vi "Data Sensor.vi"(0 "VISA resource name":refnum<visa-resource-name>, 5 "Input (0:All)":u16(ring) items=["All Inputs", "1", "2", "3", "4", "5", "6", "7", "8"], 7 "Data Source (0:Kelvin)":u16(ring) items=["Kelvin", "Celsius", "Sensor Units", "Linear Data"], 11 "error in (no error)":errorcluster) -> (1 "Input 1":dbl min=-9999.9 max=9999.9 step=0.0001 format="%.4f", 2 "Input 2":dbl min=-9999.9 max=9999.9 step=0.0001 format="%.4f", 3 "Input 3":dbl min=-9999.9 max=9999.9 step=0.0001 format="%.4f", 4 "VISA resource name out":refnum<visa-resource-name>, 6 "Input 4":dbl min=-9999.9 max=9999.9 step=0.0001 format="%.4f", 8 "Input 5":dbl min=-9999.9 max=9999.9 step=0.0001 format="%.4f", 10 "Input 6":dbl min=-9999.9 max=9999.9 step=0.0001 format="%.4f", 13 "Input 8":dbl min=-9999.9 max=9999.9 step=0.0001 format="%.4f", 14 "Input 7":dbl min=-9999.9 max=9999.9 step=0.0001 format="%.4f", 15 "error out":errorcluster)   [LabVIEW 2017, in "Lake Shore Cryotronics 218.lvlib"]
doc: "This VI reads the sensor data from all 8 of the 218's inputs. All inputs may be read with one query, this should be done to achieve the maximum reading rate of 16 rdgs/sec of all inputs. This VI can also be configured to read only one input at a time."
uses:
  Lake Shore Cryotronics 218.lvlib
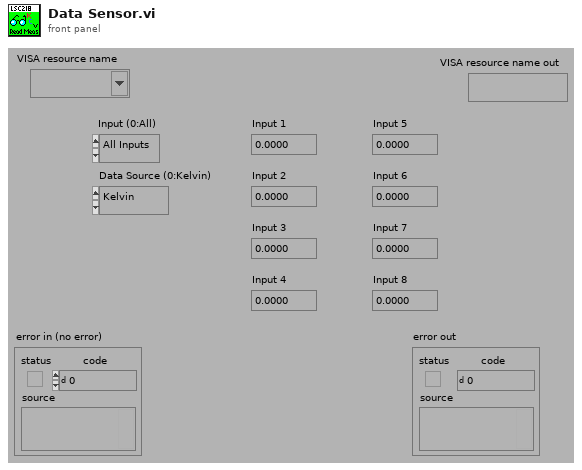
[diagram p1: front panel]
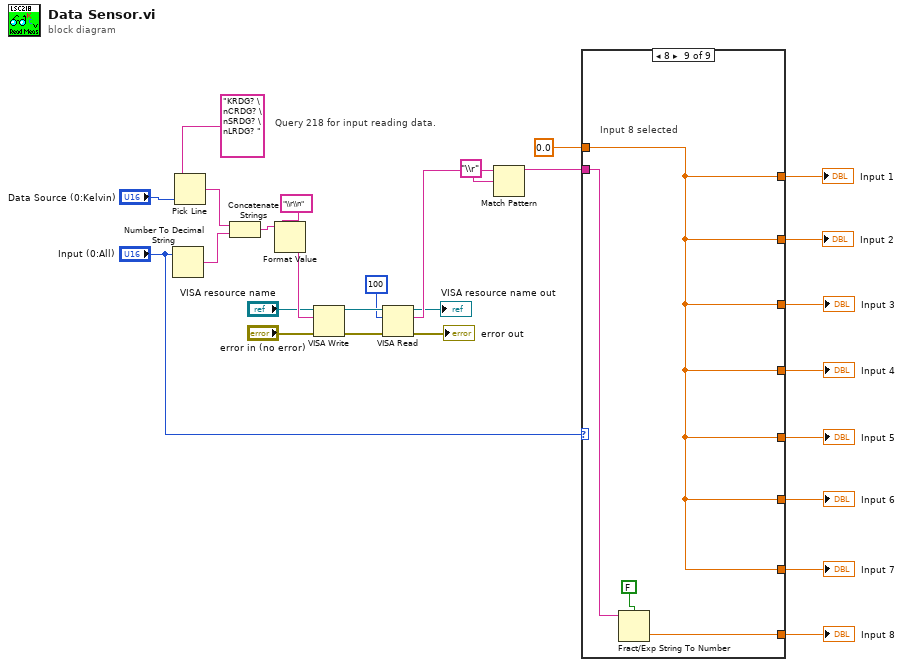
[diagram p0: block diagram]
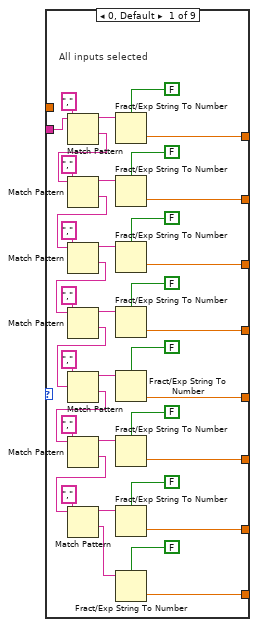
[diagram p2: hidden frame]
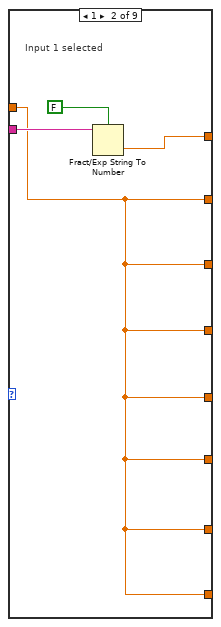
[diagram p3: hidden frame]
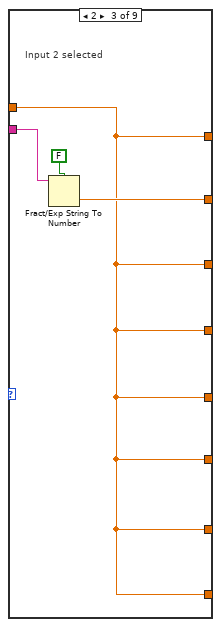
[diagram p4: hidden frame]
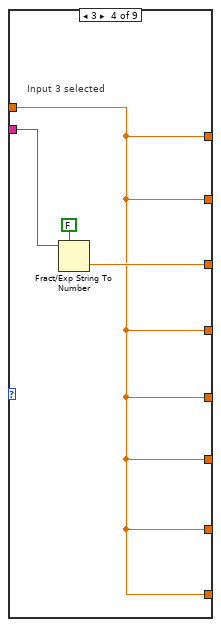
[diagram p5: hidden frame]
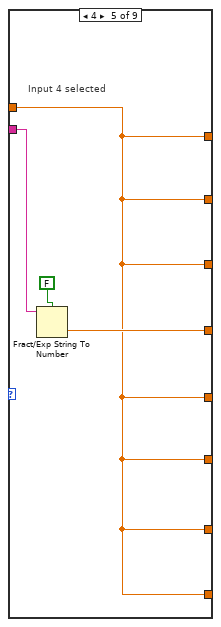
[diagram p6: hidden frame]
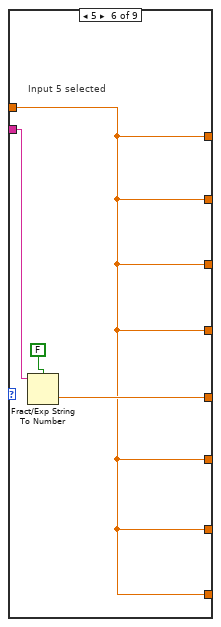
[diagram p7: hidden frame]
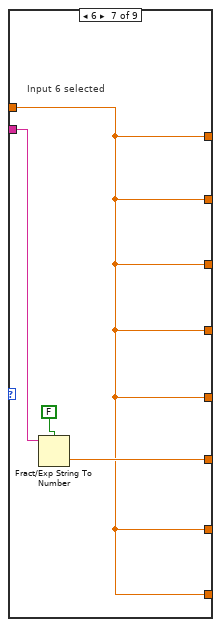
[diagram p8: hidden frame]
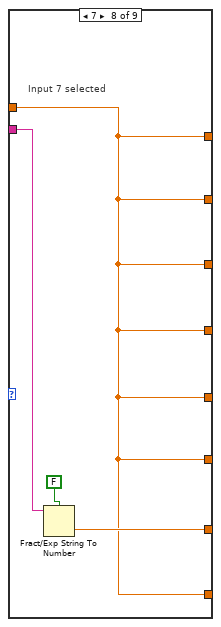
[diagram p9: hidden frame]
diagram:
  # "Query 218 for input reading data."
  n1 = Number To Decimal String(number="Input (0:All)") -> (decimal integer string=w19:string)  [unwired: 1 in]
  n2 = Pick Line(multi-line string="KRDG? \nCRDG? \nSRDG? \nLRDG? ", line index="Data Source (0:Kelvin)") -> (output string=w20:string)  [unwired: 1 in]
  n3 = Concatenate Strings(w20, w19) -> (w5:string)
  n4 = Format Value(string ("")=w5, format string="\\r\\n") -> (output string=w6:string)  [unwired: 1 in]
  n5 = VISA Write(VISA resource name="VISA resource name", write buffer=w6, error in (no error)="error in (no error)") -> (VISA resource name out=w27:refnum<visa-resource-name>, error out=w26:errorcluster)  [unwired: 1 out]
  n6 = VISA Read(VISA resource name=w27, byte count=100, error in (no error)=w26) -> (VISA resource name out=→"VISA resource name out":refnum<visa-resource-name>, read buffer=w24:string, error out=→"error out":errorcluster)  [unwired: 1 out]
  n7 = Match Pattern(string=w24, regular expression="\\r") -> (before substring=w17:string)  [unwired: 1 in, 3 out]
  n8 = case shown="8" "Input (0:All)" {
    tunnel: w17 -> [w65 w69 w73 w77 w81 w85 w89 w93 w97]
    tunnel: [w62 w68 w71 w75 w79 w83 w87 w91 w95] -> w16
    tunnel: [w58 w67 w72 w75 w79 w83 w87 w91 w95] -> w15
    tunnel: [w54 w67 w71 w76 w79 w83 w87 w91 w95] -> w14
    tunnel: [w50 w67 w71 w75 w80 w83 w87 w91 w95] -> w13
    tunnel: [w40 w67 w71 w75 w79 w84 w87 w91 w95] -> w12
    tunnel: [w39 w67 w71 w75 w79 w83 w88 w91 w95] -> w11
    tunnel: [w38 w67 w71 w75 w79 w83 w87 w92 w95] -> w10
    tunnel: [w37 w67 w71 w75 w79 w83 w87 w91 w96] -> w9
    tunnel: 0.0 -> [_ w67 w71 w75 w79 w83 w87 w91 w95]
    frame 0, Default {
      # "All inputs selected"
      n9 = Match Pattern(string=w65, regular expression=",") -> (before substring=w63:string, after substring=w59:string)  [unwired: 1 in, 2 out]
      n10 = Match Pattern(string=w59, regular expression=",") -> (before substring=w61:string, after substring=w55:string)  [unwired: 1 in, 2 out]
      n11 = Match Pattern(string=w55, regular expression=",") -> (before substring=w56:string, after substring=w51:string)  [unwired: 1 in, 2 out]
      n12 = Match Pattern(string=w51, regular expression=",") -> (before substring=w53:string, after substring=w43:string)  [unwired: 1 in, 2 out]
      n13 = Match Pattern(string=w43, regular expression=",") -> (before substring=w48:string, after substring=w42:string)  [unwired: 1 in, 2 out]
      n14 = Match Pattern(string=w42, regular expression=",") -> (before substring=w47:string, after substring=w41:string)  [unwired: 1 in, 2 out]
      n15 = Match Pattern(string=w41, regular expression=",") -> (before substring=w45:string, after substring=w36:string)  [unwired: 1 in, 2 out]
      n16 = Fract/Exp String To Number(use system decimal point (T)=FALSE, string=w63) -> (number=w62:dbl)  [unwired: 2 in, 1 out]
      n17 = Fract/Exp String To Number(use system decimal point (T)=FALSE, string=w61) -> (number=w58:dbl)  [unwired: 2 in, 1 out]
      n18 = Fract/Exp String To Number(use system decimal point (T)=FALSE, string=w56) -> (number=w54:dbl)  [unwired: 2 in, 1 out]
      n19 = Fract/Exp String To Number(use system decimal point (T)=FALSE, string=w53) -> (number=w50:dbl)  [unwired: 2 in, 1 out]
      n20 = Fract/Exp String To Number(use system decimal point (T)=FALSE, string=w48) -> (number=w40:dbl)  [unwired: 2 in, 1 out]
      n21 = Fract/Exp String To Number(use system decimal point (T)=FALSE, string=w47) -> (number=w39:dbl)  [unwired: 2 in, 1 out]
      n22 = Fract/Exp String To Number(use system decimal point (T)=FALSE, string=w45) -> (number=w38:dbl)  [unwired: 2 in, 1 out]
      n23 = Fract/Exp String To Number(use system decimal point (T)=FALSE, string=w36) -> (number=w37:dbl)  [unwired: 2 in, 1 out]
    }
    frame 1 {
      # "Input 1 selected"
      n24 = Fract/Exp String To Number(use system decimal point (T)=FALSE, string=w69) -> (number=w68:dbl)  [unwired: 2 in, 1 out]
    }
    frame 2 {
      # "Input 2 selected"
      n25 = Fract/Exp String To Number(use system decimal point (T)=FALSE, string=w73) -> (number=w72:dbl)  [unwired: 2 in, 1 out]
    }
    frame 3 {
      # "Input 3 selected"
      n26 = Fract/Exp String To Number(use system decimal point (T)=FALSE, string=w77) -> (number=w76:dbl)  [unwired: 2 in, 1 out]
    }
    frame 4 {
      # "Input 4 selected"
      n27 = Fract/Exp String To Number(use system decimal point (T)=FALSE, string=w81) -> (number=w80:dbl)  [unwired: 2 in, 1 out]
    }
    frame 5 {
      # "Input 5 selected"
      n28 = Fract/Exp String To Number(use system decimal point (T)=FALSE, string=w85) -> (number=w84:dbl)  [unwired: 2 in, 1 out]
    }
    frame 6 {
      # "Input 6 selected"
      n29 = Fract/Exp String To Number(use system decimal point (T)=FALSE, string=w89) -> (number=w88:dbl)  [unwired: 2 in, 1 out]
    }
    frame 7 {
      # "Input 7 selected"
      n30 = Fract/Exp String To Number(use system decimal point (T)=FALSE, string=w93) -> (number=w92:dbl)  [unwired: 2 in, 1 out]
    }
    frame 8 {
      # "Input 8 selected"
      n31 = Fract/Exp String To Number(use system decimal point (T)=FALSE, string=w97) -> (number=w96:dbl)  [unwired: 2 in, 1 out]
    }
  }
  "Input 1" <- w16
  "Input 2" <- w15
  "Input 3" <- w14
  "Input 4" <- w13
  "Input 5" <- w12
  "Input 6" <- w11
  "Input 7" <- w10
  "Input 8" <- w9
